vi "PRL Access Buffer Writer.vi"(5 "Write?":bool, 7 "Initialize?":bool) -> (0 "Lost Data?":bool, 1 "Activity Monitor":dbl, 2 "Refresh?":bool, 3 "Writing?":bool)   [LabVIEW 2018, in "S3DK.lvlib" / "PMU Recorder Light.lvlib"]
doc: "Reads data from the PRL Data Queue, and writes it to the Access Buffer."
uses:
  PMU Recorder Light.lvlib
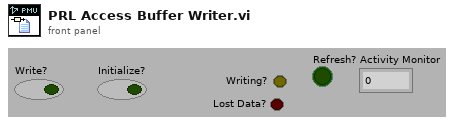
[diagram p1: front panel]
types:
  T1 = cluster{"Timestamp Values":timestamp[], "Phasor Values":csg[][], "Analog Values":sgl[][], "Digital Values":bool[][], "System Data Buffer":sgl[][]}
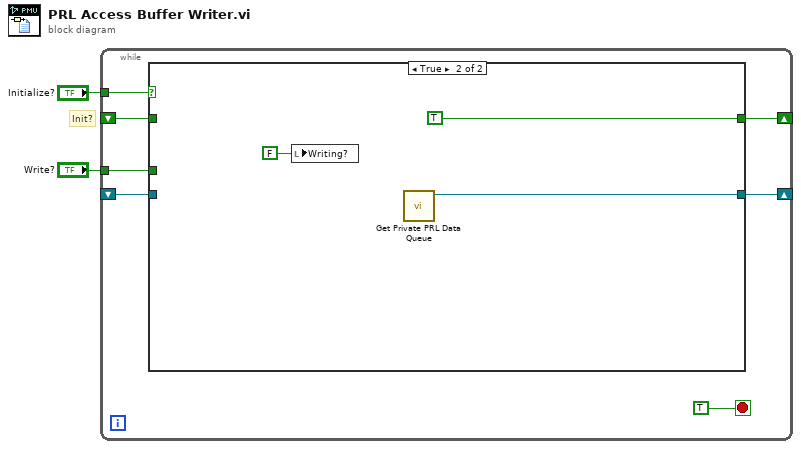
[diagram p0: block diagram]
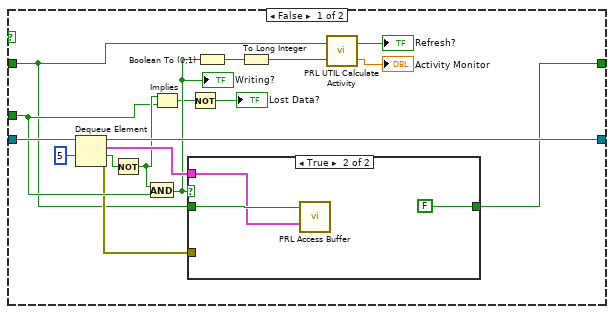
[diagram p2: hidden frame]
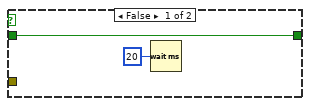
[diagram p3: hidden frame]
diagram:
  # "Init?"
  n1 = while {
    tunnel: "Initialize?" -> [w9]
    shift-right: [w8] -> _
    shift-left: _ -> [w7]
    shift-right: [w4] -> _
    shift-left: _ -> [w5]
    tunnel: "Write?" -> [w3]
    stop <- TRUE stop-if-true
    n2 = case shown="True" w9 {
      tunnel: [w25 w32] -> w8
      tunnel: w7 -> [w26 _]
      tunnel: w5 -> [w13 _]
      tunnel: [w20 TRUE ("Data?")] -> w4
      tunnel: w3 -> [w15 _]
      frame False {
        n3 = Dequeue Element(queue=w26, timeout in ms (-1)=5) -> (queue out=w25:refnum<queue>, element=w23:T1, timed out?=w22:bool, error out=w14:errorcluster)  [unwired: 1 in]
        n4 = Not(x=w22) -> (.not. x?=w16:bool)
        n5 = And(x=w16, y=w15) -> (x .and. y?=w19:bool)
        "Writing?" <- w19
        n6 = Implies(1:w15, 2:w16) -> (0:w18:bool)
        n7 = case shown="True" w19 {
          tunnel: w23 -> [_ w29]
          tunnel: w13 -> [w28 w30]
          tunnel: [w28 FALSE ("Data?")] -> w20
          tunnel: w14 -> [_ _]
          frame False {
            n8 = Wait (ms)(milliseconds to wait=u32 20) -> ()  [unwired: 1 out]
          }
          frame True {
            n9 = call "PRL Access Buffer.vi"("PMU Data Buffers"=w29, "Initialize Buffer?"=w30) -> ()  [unwired: 3 in, 7 out]
          }
        }
        n10 = Not(x=w18) -> (.not. x?=→"Lost Data?":bool)
        n11 = Boolean To (0,1)(Boolean=w19) -> (0, 1=w21:i16)
        n12 = To Long Integer(number=w21) -> (32bit integer=w12:i32)
        n13 = call "PRL UTIL Calculate Activity.vi"("Data Indicator"=w12, "Init?"=w13) -> ("Activity Monitor"=→"Activity Monitor":dbl, "Refresh?"=→"Refresh?":bool)
      }
      frame True {
        n14 = local write "Writing?"(FALSE ("Data?")) -> ()
        n15 = call "Get Private PRL Data Queue.vi"() -> ("PRL Data Queue"=w32:refnum<queue>)  [unwired: 11 in]
      }
    }
  }
